vi "num.vi"(9 "枚举":enum16{"write", "read"}(ring)=enum."read", 11 "num":i32) -> (3 "num":i32)   [LabVIEW 2018]
doc: "储存文件时的轮数标号，第n个文件"
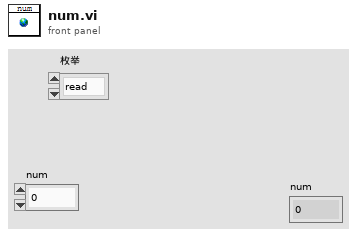
[diagram p1: front panel]
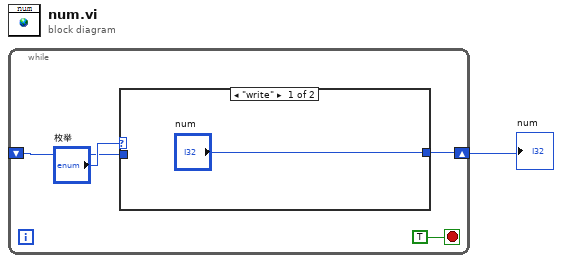
[diagram p0: block diagram]
diagram:
  n1 = while {
    shift-right: [w3] -> w1
    shift-left: _ -> [w2]
    stop <- TRUE stop-if-true
    n2 = case shown="\"write\"" "枚举" {
      tunnel: ["num" w7] -> w3
      tunnel: w2 -> [_ w7]
      frame "write" {
      }
      frame "read", Default {
      }
    }
  }
  "num" <- w1
